vi "Global - pR netw comm.vi"() -> ()   [LabVIEW 2014]
panel:
  in  "Pointer IP add":string="127.0.0.1"
  out "Pointer ON":bool
  in  "Disable pR loopback":bool
  out "pR netw Error?":bool
  out "pR netw Connected?":bool
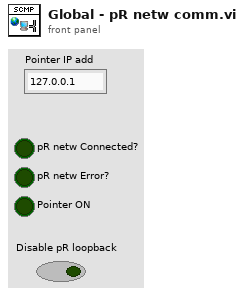
[diagram p1: front panel]
diagram:
